vi "Write IProjectItemFactory.vi"(10 "IProjectItemFactory":refnum<class "IProjectItemFactory.lvclass">, 11 "ProjectItem in":refnum<class "ProjectItem.lvclass">) -> (3 "ProjectItem out":refnum<class "ProjectItem.lvclass">)   [LabVIEW 2016, in "ProjectItem.lvclass"]
uses:
  ProjectItem.lvclass
  IProjectItemFactory/IProjectItemFactory.lvclass
  ProjectItem.lvclass/ProjectItem.ctl
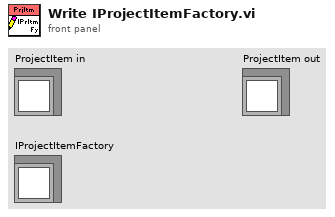
[diagram p1: front panel]
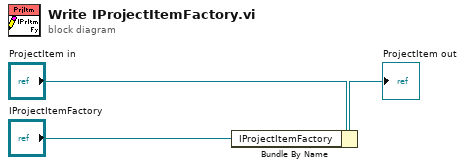
[diagram p0: block diagram]
diagram:
  n1 = Bundle By Name(cluster="ProjectItem in", "IProjectItemFactory"="IProjectItemFactory") -> (→"ProjectItem out":refnum<class "ProjectItem.lvclass">)
